vi "get_credy_path.vi"() -> (1 "appended path":path)   [LabVIEW 2019]
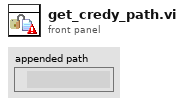
[diagram p1: front panel]
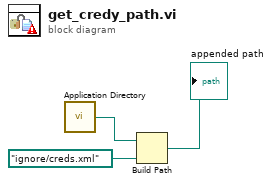
[diagram p0: block diagram]
diagram:
  n1 = call <vilib>:"Application Directory.vi"() -> ("Application Directory"=w1:path)
  n2 = Build Path(base path=w1, name or relative path=path "ignore/creds.xml" ("XML File Path")) -> (appended path=→"appended path":path)
